vi "Teleop.vi"(10 "Match Info":T1={"Autonomous Elapsed Seconds"=0.0, "TeleOp Elapsed Seconds"=0.0, "Disabled Elapsed Seconds"=0.0, "Visited Autonomous"=FALSE, "Visited TeleOp"=FALSE, "Visited Disabled"=FALSE, "Autonomous Settings"={"Autonomous Style"=enum."Independent", "VI Refnum"=refnum}}, 11 "Call Context":T2) -> ()   [LabVIEW 2016]
doc: "This VI is called for each TeleOp packet received from the DS where the robot is not disabled. It is often used to read from the joysticks and update I/O or to update setpoints for timed control loops. It should complete and return within 20 milliseconds or it may miss DS packets."
uses:
  <vilib>/Rock Robotics/WPI/DriverStation/WPI_DriverStationDerivedRobotMode.ctl
  <vilib>/Rock Robotics/WPI/DriverStation/WPI_DriverStationMatch Info.ctl
  <vilib>/Rock Robotics/WPI/Solenoid/WPI_SolenoidValue.ctl
  <vilib>/Rock Robotics/WPI/Utilities/WPI_GetSetVariantRefNum.vi
  <vilib>/Rock Robotics/Network Tables/NT Write Boolean Array.vi
  <vilib>/Rock Robotics/Network Tables/NT Write Numeric Array.vi
  <vilib>/Rock Robotics/Network Tables/NT Read Boolean.vi
  <vilib>/Rock Robotics/Network Tables/NT Read Number.vi
  <vilib>/Rock Robotics/WPI/Solenoid/WPI_SolenoidSetEnum.vi
panel:
  out "Sample Slider 0":dbl(slide) scale=0.0..5.0
  out "Sample Boolean 1":bool
  out "Sample Boolean 0":bool
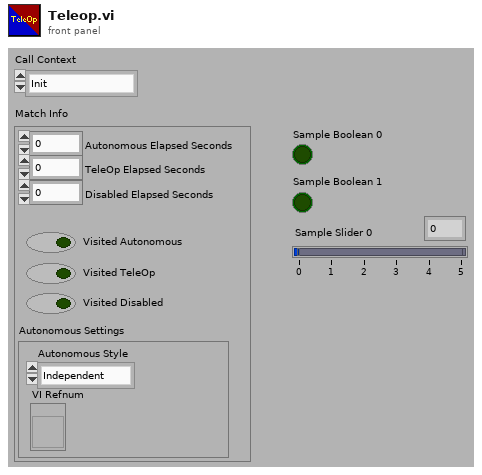
[diagram p1: front panel]
types:
  T1 = typedef "WPI_DriverStationMatch Info.ctl" = cluster{"Autonomous Elapsed Seconds":dbl, "TeleOp Elapsed Seconds":dbl, "Disabled Elapsed Seconds":dbl, "Visited Autonomous":bool, "Visited TeleOp":bool, "Visited Disabled":bool, "Autonomous Settings":cluster{"Autonomous Style":enum16{"Iterative", "Independent"}, "VI Refnum":refnum<vi>}}
  T2 = typedef "WPI_DriverStationDerivedRobotMode.ctl" = enum16{"Init", "Execute", "Stop"}
  T3 = typedef "WPI_JoystickDevRef.ctl" = cluster{"Device":T4}
  T4 = typedef "WPI_JoystickDeviceEnum.ctl" = enum16{"USB 0", "USB 1", "USB 2", "USB 3", "USB 4", "USB 5"}
  T5 = typedef "WPI_RobotDriveDevRef.ctl" = cluster{"DevStatus":errorcluster, "Motors[]":T6[], "Square Inputs":bool, "Max Output":dbl}
  T6 = typedef "WPI_MotorControlDeviceRef.ctl" = cluster{"DeviceStatus":errorcluster, "Type":T7, "PWM":cluster{"PWM Channel":T8, "DeadBand":T9}, "CAN":cluster{"Device Number":u8, "SetOutput VI Ref":variant, "GetOutput VI Ref":variant, "Enable VI Ref":variant, "Disable VI Ref":variant, "Data":variant}, "Invert":bool}
  T7 = typedef "WPI_MotorControlType.ctl" = enum16{"PWM", "CAN"}
  T8 = typedef "FPGA_DIOPWMChannel.ctl" = enum8{"PWM 0", "PWM 1", "PWM 2", "PWM 3", "PWM 4", "PWM 5", "PWM 6", "PWM 7", "PWM 8", "PWM 9", "PWM MXP 0", "PWM MXP 1", "PWM MXP 2", "PWM MXP 3", "PWM MXP 4", "PWM MXP 5", "PWM MXP 6", "PWM MXP 7", "PWM MXP 8", "PWM MXP 9", "Invalid"}
  T9 = typedef "WPI_PWMDeadband.ctl" = cluster{"Name":string, "maxPositivePwm":i32, "minPositivePwm":i32, "centerPwm":i32, "maxNegativePwm":i32, "minNegativePwm":i32, "angularRange":u16}
  T10 = cluster{"Buttons[0]":bool, "Buttons[1]":bool, "Buttons[2]":bool, "Buttons[3]":bool, "Buttons[4]":bool, "Buttons[5]":bool, "Buttons[6]":bool, "Buttons[7]":bool, "Buttons[8]":bool}
  T11 = typedef "WPI_SolenoidValue.ctl" = enum16{"Off", "On", "Forward", "Reverse"}
  T12 = typedef "WPI_SolenoidDevRef.ctl" = cluster{"DevStatus":errorcluster, "Pneumatics Control Module":u8, "Forward Solenoid Channel":T13, "Reverse Solenoid Channel":T13}
  T13 = typedef "WPI_SolenoidChannel.ctl" = enum8{"Solenoid 0", "Solenoid 1", "Solenoid 2", "Solenoid 3", "Solenoid 4", "Solenoid 5", "Solenoid 6", "Solenoid 7", "Invalid"}
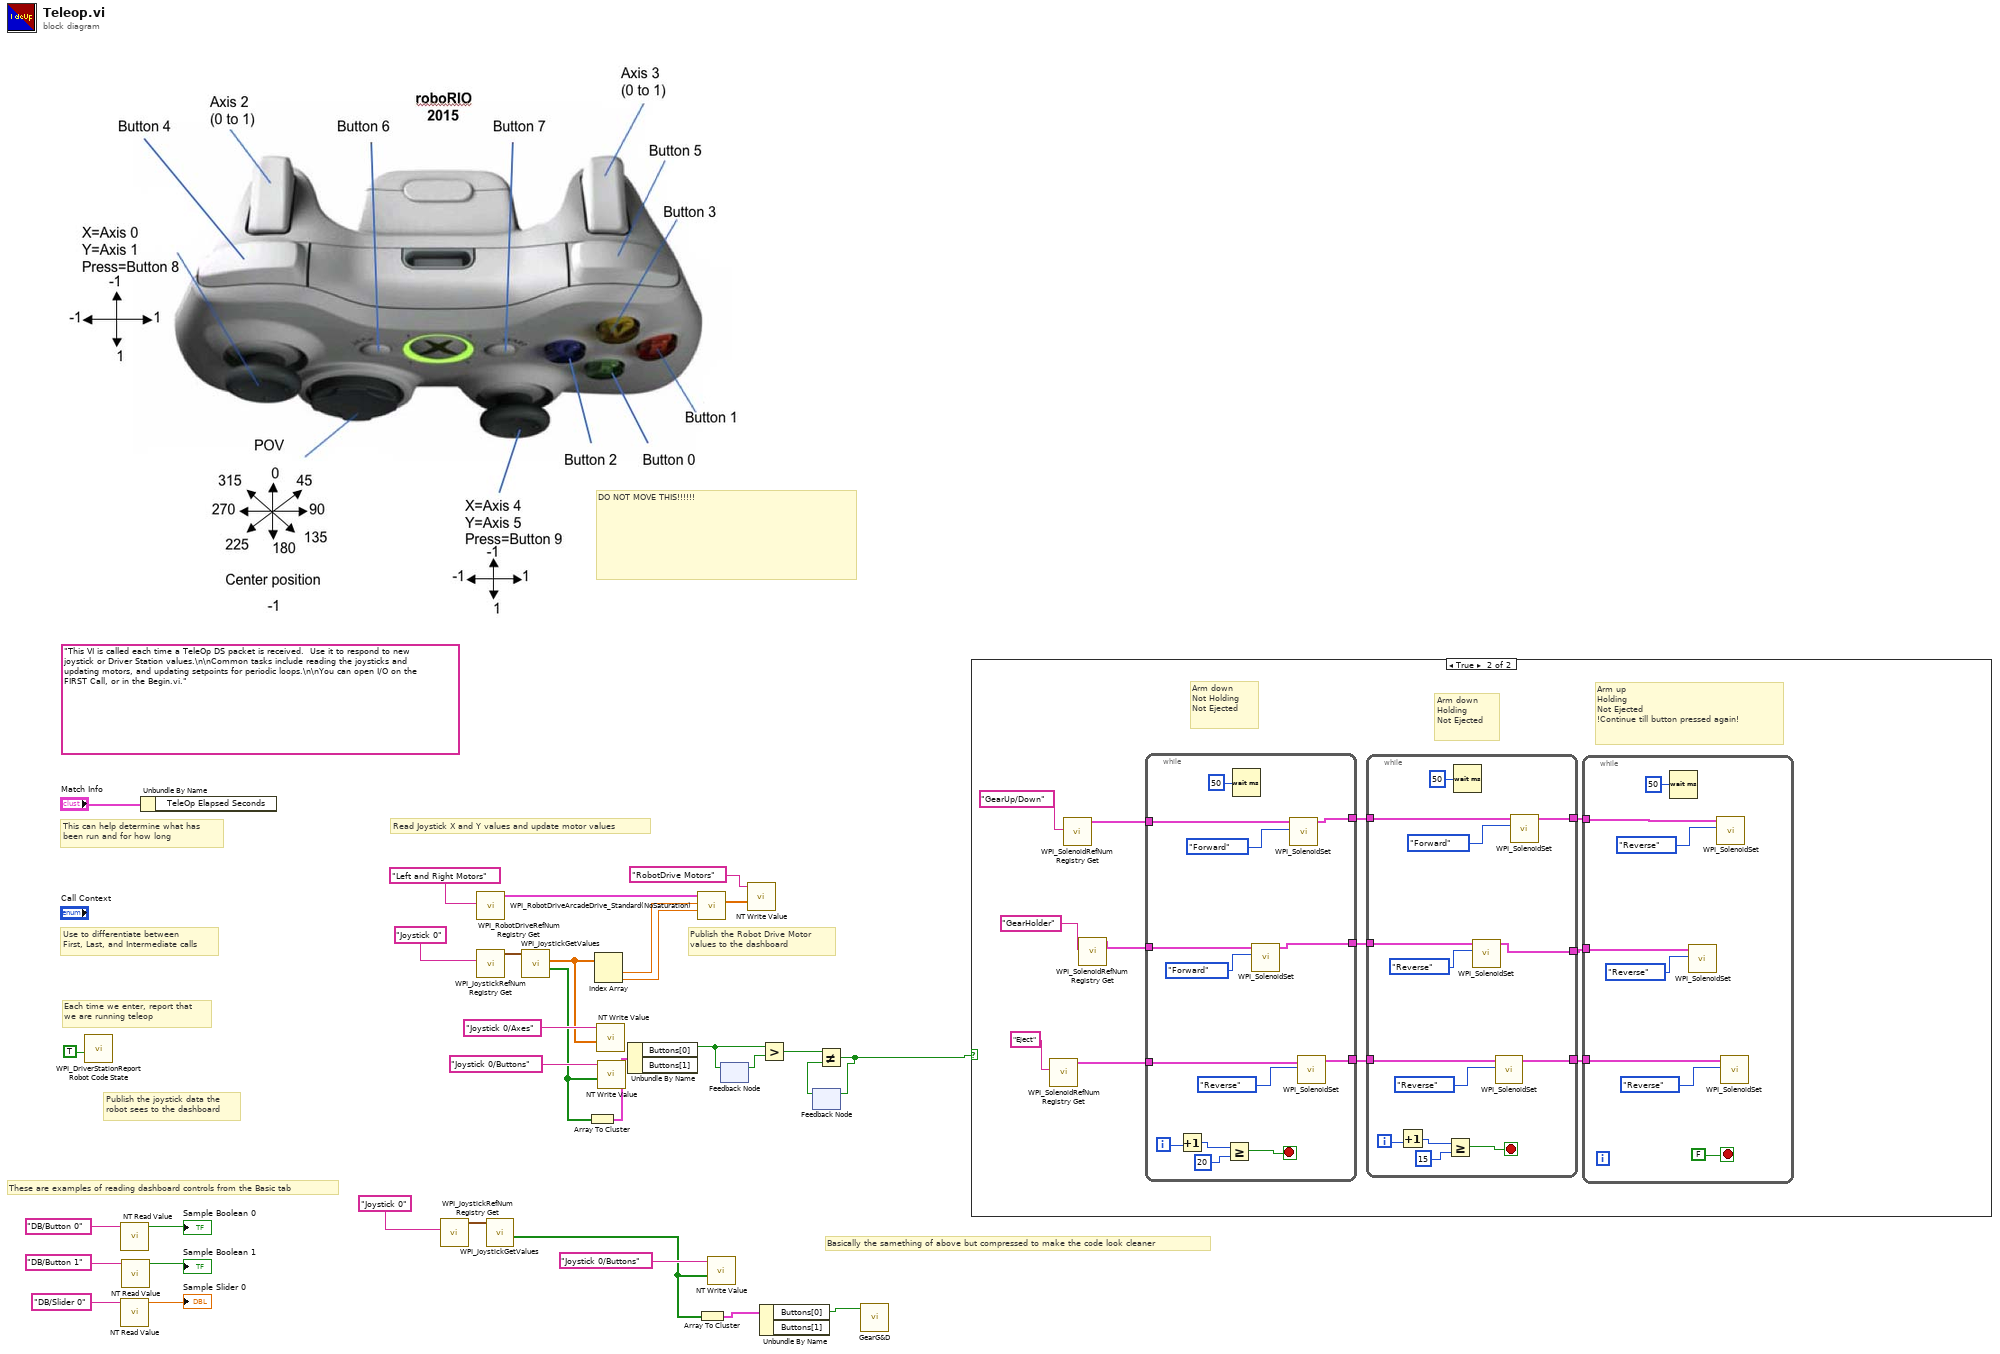
[diagram p0: block diagram]
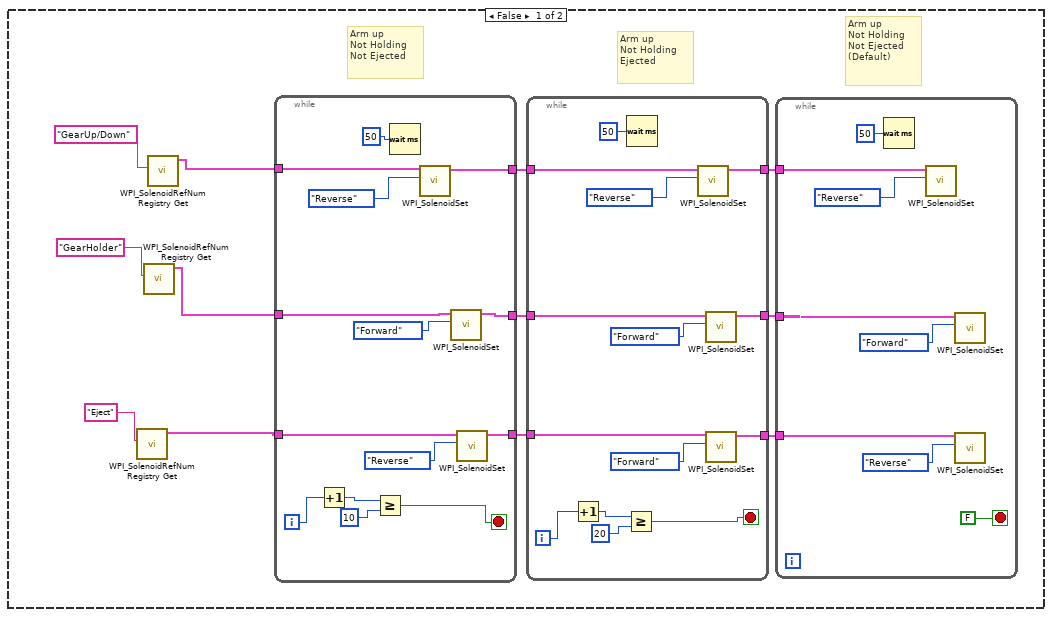
[diagram p2: hidden frame]
diagram:
  (unwired) "This VI is called each time a TeleOp DS packet is received.  Use it to respond to new joystick or Driver Station values.\n\nCommon tasks include reading the joysticks and updating motors, and updating setpoints for periodic loops.\n\nYou can open I/O on the FIRST Call, or in the Begin.vi."
  # "DO NOT MOVE THIS!!!!!!"
  # "Basically the samething of above but compressed to make the code look cleaner"
  # "These are examples of reading dashboard controls from the Basic tab"
  # "Publish the Robot Drive Motor\nvalues to the dashboard"
  # "Publish the joystick data the\nrobot sees to the dashboard"
  # "Each time we enter, report that\nwe are running teleop"
  # "Use to differentiate between\nFirst, Last, and Intermediate calls"
  # "This can help determine what has\nbeen run and for how long"
  # "Read Joystick X and Y values and update motor values"
  n1 = call <vilib>:"WPI_DriverStationReport Robot Code State.vi"("TeleOp"=TRUE ("Autonomous")) -> ()  [unwired: 10 in, 1 out]
  n2 = call-poly <vilib>:"NT Read Value.vi"("Name"="DB/Button 0" ("refnum name")) -> ("Boolean"=→"Sample Boolean 0":bool)  [unwired: 9 in, 1 out]
  n3 = call-poly <vilib>:"NT Read Value.vi"("Name"="DB/Slider 0" ("refnum name")) -> ("Numeric"=→"Sample Slider 0":dbl)  [unwired: 9 in, 1 out]
  n4 = call-poly <vilib>:"NT Read Value.vi"("Name"="DB/Button 1" ("refnum name")) -> ("Boolean"=→"Sample Boolean 1":bool)  [unwired: 9 in, 1 out]
  n5 = Unbundle By Name("Match Info") -> ()  [unwired: 1 out]
  n6 = call <vilib>:"WPI_JoystickRefNum Registry Get.vi"("refnum name"="Joystick 0") -> ("JoystickDevRef"=w6:T3)  [unwired: 1 in, 9 out]
  n7 = call <vilib>:"WPI_RobotDriveRefNum Registry Get.vi"("refnum name"="Left and Right Motors") -> ("RobotDriveDevRef"=w30:T5)  [unwired: 1 in, 9 out]
  n8 = call <vilib>:"WPI_JoystickRefNum Registry Get.vi"("refnum name"="Joystick 0") -> ("JoystickDevRef"=w27:T3)  [unwired: 1 in, 9 out]
  n9 = call <vilib>:"WPI_JoystickGetValues.vi"("JoystickDevRef"=w6) -> ("Buttons"=w4:bool[])  [unwired: 6 in, 4 out]
  n10 = call <vilib>:"WPI_JoystickGetValues.vi"("JoystickDevRef"=w27) -> ("Buttons"=w13:bool[], "Axes"=w22:dbl[])  [unwired: 6 in, 3 out]
  n11 = Array To Cluster(array=w13) -> (cluster=w12:T10)
  n12 = Index Array(array=w22) -> (element #1=w29:dbl, element #2=w25:dbl)  [unwired: 2 in]
  n13 = call-poly <vilib>:"NT Write Value.vi"("Numeric Array"=w22, "Name"="Joystick 0/Axes") -> ()  [unwired: 9 in, 1 out]
  n14 = call-poly <vilib>:"NT Write Value.vi"("Boolean Array"=w13, "Name"="Joystick 0/Buttons") -> ()  [unwired: 9 in, 1 out]
  n15 = Unbundle By Name(w12) -> ("Buttons[0]"=w10:bool)  [unwired: 1 out]
  n16 = call <vilib>:"WPI_RobotDriveArcadeDrive_Standard(NoSaturation).vi"("Y axis value"=w25, "X axis value"=w29, "RobotDriveDevRef"=w30) -> ("Motor Values"=w15:dbl[])  [unwired: 1 in, 7 out]
  n17 = Array To Cluster(array=w4) -> (cluster=w3:T10)
  n18 = call-poly <vilib>:"NT Write Value.vi"("Boolean Array"=w4, "Name"="Joystick 0/Buttons") -> ()  [unwired: 9 in, 1 out]
  n19 = feedback-in #1(w10) -> ()
  n20 = feedback #1() -> (w9:bool)  [unwired: 1 in]
  n21 = call-poly <vilib>:"NT Write Value.vi"("Numeric Array"=w15, "Name"="RobotDrive Motors") -> ()  [unwired: 9 in, 1 out]
  n22 = Unbundle By Name(w3) -> ("Buttons[0]"=w2:bool)  [unwired: 1 out]
  n23 = Greater?(x=w10, y=w9) -> (0:w11:bool)
  n24 = feedback #2() -> (w8:bool)  [unwired: 1 in]
  n25 = Not Equal?(x=w11, y=w8) -> (x != y?=w1:bool)
  n26 = feedback-in #2(w1) -> ()
  n27 = call "GearG&D.vi"("Grab"=w2) -> ()  [unwired: 2 in]
  n28 = case shown="True" w1 {
    frame False {
      # "Arm up\nNot Holding\nNot Ejected\n(Default)"
      # "Arm up\nNot Holding\nEjected"
      # "Arm up\nNot Holding\nNot Ejected"
      n29 = call <vilib>:"WPI_SolenoidRefNum Registry Get.vi"("refnum name"="Eject") -> ("SolenoidDevRef"=w33:T12)  [unwired: 9 in, 1 out]
      n30 = call <vilib>:"WPI_SolenoidRefNum Registry Get.vi"("refnum name"="GearHolder") -> ("SolenoidDevRef"=w34:T12)  [unwired: 9 in, 1 out]
      n31 = call <vilib>:"WPI_SolenoidRefNum Registry Get.vi"("refnum name"="GearUp/Down") -> ("SolenoidDevRef"=w35:T12)  [unwired: 9 in, 1 out]
      n32 = while {
        tunnel: [w74] -> w41
        tunnel: [w73] -> w40
        tunnel: w34 -> [w71]
        tunnel: w33 -> [w70]
        tunnel: w35 -> [w68]
        tunnel: [w67] -> w37
        i -> [w76]
        stop <- w75 stop-if-true
        n33 = Increment(x=w76) -> (x+1=w78:i32)
        n34 = Greater Or Equal?(x=w78, y=10) -> (x >= y?=w75:bool)
        n35 = Wait (ms)(milliseconds to wait=u32 50) -> ()  [unwired: 1 out]
        n36 = call-poly <vilib>:"WPI_SolenoidSet.vi"("Value"=WPI_SolenoidValue."Reverse", "SolenoidDevRef"=w68) -> ("SolenoidDevRef"=w67:T12)  [unwired: 8 in, 1 out]
        n37 = call-poly <vilib>:"WPI_SolenoidSet.vi"("Value"=WPI_SolenoidValue."Forward", "SolenoidDevRef"=w71) -> ("SolenoidDevRef"=w73:T12)  [unwired: 8 in, 1 out]
        n38 = call-poly <vilib>:"WPI_SolenoidSet.vi"("Value"=WPI_SolenoidValue."Reverse", "SolenoidDevRef"=w70) -> ("SolenoidDevRef"=w74:T12)  [unwired: 8 in, 1 out]
      }
      n39 = while {
        tunnel: w41 -> [w64]
        tunnel: w40 -> [w63]
        tunnel: [w58] -> w39
        tunnel: [w57] -> w38
        tunnel: w37 -> [w54]
        tunnel: [w53] -> w36
        i -> [w60]
        stop <- w59 stop-if-true
        n40 = Increment(x=w60) -> (x+1=w62:i32)
        n41 = Greater Or Equal?(x=w62, y=20) -> (x >= y?=w59:bool)
        n42 = Wait (ms)(milliseconds to wait=u32 50) -> ()  [unwired: 1 out]
        n43 = call-poly <vilib>:"WPI_SolenoidSet.vi"("Value"=WPI_SolenoidValue."Reverse", "SolenoidDevRef"=w54) -> ("SolenoidDevRef"=w53:T12)  [unwired: 8 in, 1 out]
        n44 = call-poly <vilib>:"WPI_SolenoidSet.vi"("Value"=WPI_SolenoidValue."Forward", "SolenoidDevRef"=w63) -> ("SolenoidDevRef"=w57:T12)  [unwired: 8 in, 1 out]
        n45 = call-poly <vilib>:"WPI_SolenoidSet.vi"("Value"=WPI_SolenoidValue."Forward", "SolenoidDevRef"=w64) -> ("SolenoidDevRef"=w58:T12)  [unwired: 8 in, 1 out]
      }
      n46 = while {
        tunnel: w39 -> [w50]
        tunnel: w38 -> [w49]
        tunnel: w36 -> [w45]
        stop <- FALSE stop-if-true
        n47 = Wait (ms)(milliseconds to wait=u32 50) -> ()  [unwired: 1 out]
        n48 = call-poly <vilib>:"WPI_SolenoidSet.vi"("Value"=WPI_SolenoidValue."Reverse", "SolenoidDevRef"=w45) -> ()  [unwired: 8 in, 2 out]
        n49 = call-poly <vilib>:"WPI_SolenoidSet.vi"("Value"=WPI_SolenoidValue."Forward", "SolenoidDevRef"=w49) -> ()  [unwired: 8 in, 2 out]
        n50 = call-poly <vilib>:"WPI_SolenoidSet.vi"("Value"=WPI_SolenoidValue."Reverse", "SolenoidDevRef"=w50) -> ()  [unwired: 8 in, 2 out]
      }
    }
    frame True {
      # "Arm up\nHolding\nNot Ejected\n!Continue till button pressed again!"
      # "Arm down\nHolding\nNot Ejected"
      # "Arm down\nNot Holding\nNot Ejected"
      n51 = call <vilib>:"WPI_SolenoidRefNum Registry Get.vi"("refnum name"="Eject") -> ("SolenoidDevRef"=w83:T12)  [unwired: 9 in, 1 out]
      n52 = call <vilib>:"WPI_SolenoidRefNum Registry Get.vi"("refnum name"="GearUp/Down") -> ("SolenoidDevRef"=w91:T12)  [unwired: 9 in, 1 out]
      n53 = call <vilib>:"WPI_SolenoidRefNum Registry Get.vi"("refnum name"="GearHolder") -> ("SolenoidDevRef"=w89:T12)  [unwired: 9 in, 1 out]
      n54 = while {
        tunnel: w91 -> [w128]
        tunnel: w89 -> [w127]
        tunnel: [w119] -> w88
        tunnel: [w118] -> w87
        tunnel: w83 -> [w116]
        tunnel: [w115] -> w82
        i -> [w124]
        stop <- w121 stop-if-true
        n55 = Increment(x=w124) -> (x+1=w122:i32)
        n56 = Greater Or Equal?(x=w122, y=20) -> (x >= y?=w121:bool)
        n57 = Wait (ms)(milliseconds to wait=u32 50) -> ()  [unwired: 1 out]
        n58 = call-poly <vilib>:"WPI_SolenoidSet.vi"("Value"=WPI_SolenoidValue."Forward", "SolenoidDevRef"=w127) -> ("SolenoidDevRef"=w118:T12)  [unwired: 8 in, 1 out]
        n59 = call-poly <vilib>:"WPI_SolenoidSet.vi"("Value"=WPI_SolenoidValue."Forward", "SolenoidDevRef"=w128) -> ("SolenoidDevRef"=w119:T12)  [unwired: 8 in, 1 out]
        n60 = call-poly <vilib>:"WPI_SolenoidSet.vi"("Value"=WPI_SolenoidValue."Reverse", "SolenoidDevRef"=w116) -> ("SolenoidDevRef"=w115:T12)  [unwired: 8 in, 1 out]
      }
      n61 = while {
        tunnel: w88 -> [w114]
        tunnel: w87 -> [w113]
        tunnel: [w105] -> w86
        tunnel: [w104] -> w85
        tunnel: w82 -> [w102]
        tunnel: [w101] -> w81
        i -> [w110]
        stop <- w107 stop-if-true
        n62 = Increment(x=w110) -> (x+1=w108:i32)
        n63 = Greater Or Equal?(x=w108, y=15) -> (x >= y?=w107:bool)
        n64 = Wait (ms)(milliseconds to wait=u32 50) -> ()  [unwired: 1 out]
        n65 = call-poly <vilib>:"WPI_SolenoidSet.vi"("Value"=WPI_SolenoidValue."Reverse", "SolenoidDevRef"=w113) -> ("SolenoidDevRef"=w104:T12)  [unwired: 8 in, 1 out]
        n66 = call-poly <vilib>:"WPI_SolenoidSet.vi"("Value"=WPI_SolenoidValue."Reverse", "SolenoidDevRef"=w102) -> ("SolenoidDevRef"=w101:T12)  [unwired: 8 in, 1 out]
        n67 = call-poly <vilib>:"WPI_SolenoidSet.vi"("Value"=WPI_SolenoidValue."Forward", "SolenoidDevRef"=w114) -> ("SolenoidDevRef"=w105:T12)  [unwired: 8 in, 1 out]
      }
      n68 = while {
        tunnel: w86 -> [w100]
        tunnel: w85 -> [w99]
        tunnel: w81 -> [w94]
        stop <- FALSE stop-if-true
        n69 = Wait (ms)(milliseconds to wait=u32 50) -> ()  [unwired: 1 out]
        n70 = call-poly <vilib>:"WPI_SolenoidSet.vi"("Value"=WPI_SolenoidValue."Reverse", "SolenoidDevRef"=w99) -> ()  [unwired: 8 in, 2 out]
        n71 = call-poly <vilib>:"WPI_SolenoidSet.vi"("Value"=WPI_SolenoidValue."Reverse", "SolenoidDevRef"=w100) -> ()  [unwired: 8 in, 2 out]
        n72 = call-poly <vilib>:"WPI_SolenoidSet.vi"("Value"=WPI_SolenoidValue."Reverse", "SolenoidDevRef"=w94) -> ()  [unwired: 8 in, 2 out]
      }
    }
  }
